vi "Mod_OFDM_DeMapping.vi"(0 "FFT {X}":cdb[][](array[numeric]), 11 "error in (no error)":errorcluster, 13 "Parameters per Ofdm Symbol":T1 {"Data Source"."Data Source"."Register Initial State" format="%08x"}) -> (4 "Bits Out":i8[](array[numeric]), 15 "error out":errorcluster)   [LabVIEW 2010]
uses:
  Controls(Type_DEf)/Parameters per Ofdm Symbol.ctl
  <vilib>/AddOns/Modulation/Digital/General/MT Generate QAM System Parameters(M).vi
  <vilib>/addons/Modulation/Digital/General/MT Map QAM Symbols to Bits.vi
  <vilib>/AddOns/Modulation/Digital/General/MT Generate PSK System Parameters(M).vi
  <vilib>/addons/Modulation/Digital/General/MT Map PSK Symbols to Bits.vi
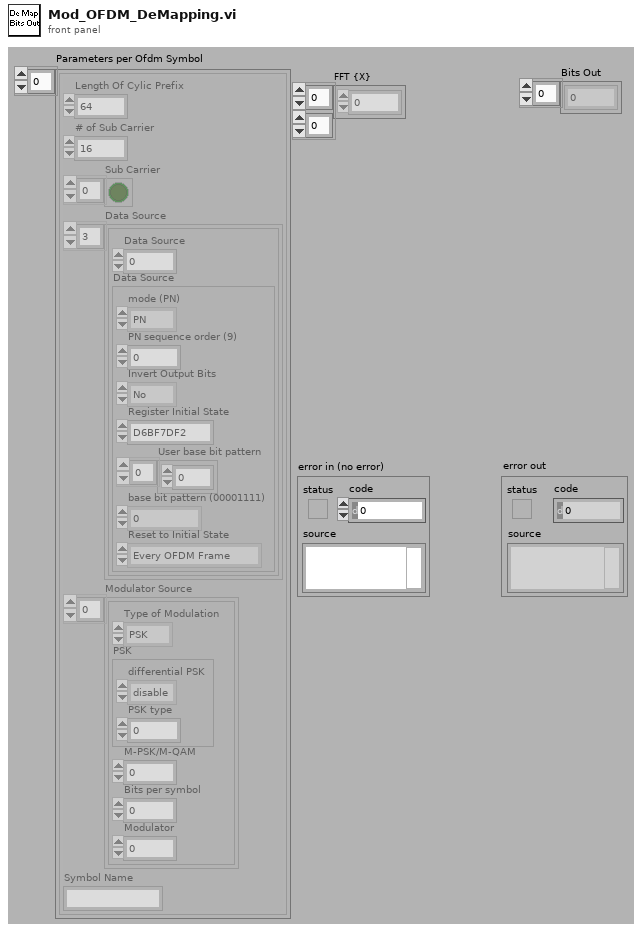
[diagram p1: front panel]
types:
  T1 = typedef "Parameters per Ofdm Symbol.ctl" = cluster{"Length Of Cylic Prefix":i32, "# of Sub Carrier":i32, "Sub Carrier":bool[], "Data Source":cluster{"Data Source":u16, "Data Source":cluster{"mode (PN)":enum16{"PN", "pattern", "user"}, "PN sequence order (9)":i32, "Invert Output Bits":enum16{"No", "Yes"}, "Register Initial State":u32, "User base bit pattern":i8[], "base bit pattern (00001111)":enum16{"0", "1", "01", "0011", "00001111"}, "Reset to Initial State":enum16{"Every OFDM Frame", "Every OFDM Symbol", "Every Sub Carrier"}}}[], "Modulator Source":cluster{"Type of Modulation":enum16{"PSK", "QAM"}, "PSK":cluster{"differential PSK":enum16{"disable", "enable"}, "PSK type":u16}, "M-PSK/M-QAM":i32, "Bits per symbol":i32, "Modulator":u16}[], "Symbol Name":string}[]
  T2 = cluster{"Type of Modulation":enum16{"PSK", "QAM"}, "PSK":cluster{"differential PSK":enum16{"disable", "enable"}, "PSK type":u16}, "M-PSK/M-QAM":i32, "Bits per symbol":i32, "Modulator":u16}[]
  T3 = cluster{"samples per symbol (16)":i32, "symbol map":cdb[]}
  T4 = cluster{"samples per symbol (16)":i32, "symbol map":cdb[], "differential PSK":enum16{"disable", "enable"}, "PSK type":u16}
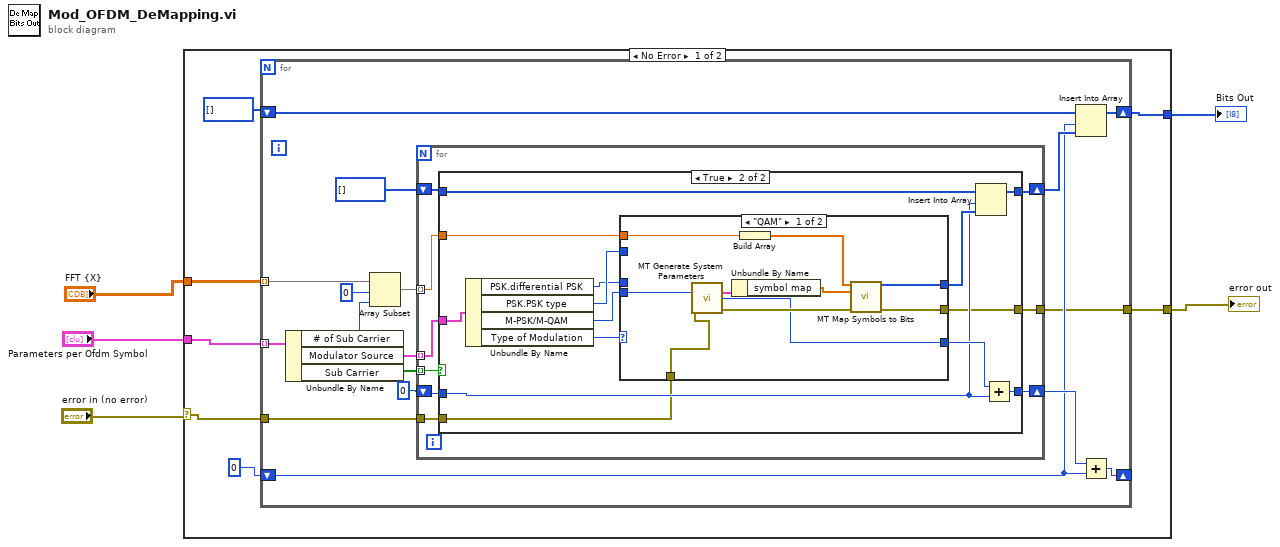
[diagram p0: block diagram]
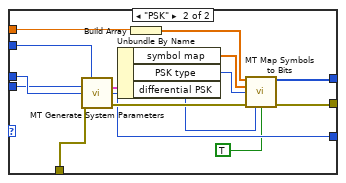
[diagram p3: hidden frame]
diagram:
  n1 = case shown="No Error" "error in (no error)" {
    selector: "error in (no error)" -> [w6 w81]
    tunnel: "Parameters per Ofdm Symbol" -> [w12 _]
    tunnel: "FFT {X}" -> [w11 _]
    tunnel: [w8 _] -> w3
    tunnel: [w7 w81] -> w2
    frame No Error {
      n2 = for {
        tunnel: w12 -> [w29] mode=indexing
        tunnel: w11 -> [w27] mode=indexing
        shift-right: [w21] -> _
        shift-left: 0 -> [w16]
        shift-right: [w19] -> w8
        shift-left: i8[] [] -> [w18]
        tunnel: w6 -> [w14]
        tunnel: [w13] -> w7
        n3 = Unbundle By Name(w29) -> ("# of Sub Carrier"=w28:i32, "Modulator Source"=w24:T2, "Sub Carrier"=w15:bool[])
        n4 = Array Subset(array=w27, index=0, length=w28) -> (w25:cdb[])
        n5 = for {
          tunnel: w25 -> [w36] mode=indexing
          tunnel: w24 -> [w37] mode=indexing
          shift-right: [w33] -> w17
          shift-left: 0 -> [w38]
          shift-right: [w34] -> w20
          shift-left: i8[] [] -> [w35]
          tunnel: w15 -> [w32] mode=indexing
          tunnel: w14 -> [w31]
          tunnel: [w30] -> w13
          n6 = case shown="True" w32 {
            tunnel: w35 -> [w41 w51]
            tunnel: w38 -> [w40 w50]
            tunnel: [w40 w49] -> w33
            tunnel: [w41 w48] -> w34
            tunnel: w37 -> [_ w47]
            tunnel: w36 -> [_ w46]
            tunnel: w31 -> [w39 w43]
            tunnel: [w39 w42] -> w30
            frame False {
            }
            frame True {
              n7 = Unbundle By Name(w47) -> ("PSK.differential PSK"=w54:enum16{"disable", "enable"}, "PSK.PSK type"=w55:u16, "M-PSK/M-QAM"=w45:i32, "Type of Modulation"=w44:enum16{"PSK", "QAM"})
              n8 = case shown="\"QAM\"" w44 {
                tunnel: w46 -> [w63 w78]
                tunnel: w45 -> [w64 w73]
                tunnel: [w61 w77] -> w53
                tunnel: [w60 w74] -> w52
                tunnel: w55 -> [_ w76]
                tunnel: w54 -> [_ w75]
                tunnel: w43 -> [w59 w72]
                tunnel: [w58 w71] -> w42
                frame "QAM" {
                  n9 = call-poly <vilib>:"MT Generate System Parameters.vi"("M-QAM (16)"=w64, "error in (no error)"=w59) -> ("QAM system parameters"=w57:T3, "bits per symbol"=w60:i32, "error out"=w65:errorcluster)  [unwired: 11 in]
                  n10 = Unbundle By Name(w57) -> ("symbol map"=w56:cdb[])
                  n11 = Build Array(w63) -> (w62:cdb[])
                  n12 = call-poly <vilib>:"MT Map Symbols to Bits.vi"("symbols"=w62, "symbol map"=w56, "error in (no error)"=w65) -> ("output bit stream"=w61:i8[], "error out"=w58:errorcluster)  [unwired: 11 in]
                }
                frame "PSK" {
                  n13 = call-poly <vilib>:"MT Generate System Parameters.vi"("PSK type"=w76, "M-PSK (4)"=w73, "differential PSK"=w75, "error in (no error)"=w72) -> ("PSK system parameters"=w70:T4, "bits per symbol"=w74:i32, "error out"=w79:errorcluster)  [unwired: 9 in]
                  n14 = Unbundle By Name(w70) -> ("symbol map"=w69:cdb[], "PSK type"=w68:u16, "differential PSK"=w67:enum16{"disable", "enable"})
                  n15 = Build Array(w78) -> (w80:cdb[])
                  n16 = call-poly <vilib>:"MT Map Symbols to Bits.vi"("symbols"=w80, "symbol map"=w69, "PSK type"=w68, "error in (no error)"=w79, "differential PSK"=w67, "reset? (T)"=TRUE) -> ("output bit stream"=w77:i8[], "error out"=w71:errorcluster)  [unwired: 8 in]
                }
              }
              n17 = Insert Into Array(array=w51, index=w50, new element=w53) -> (w48:i8[])
              n18 = Add(x=w52, y=w50) -> (x+y=w49:i32)
            }
          }
        }
        n19 = Insert Into Array(array=w18, index=w16, new element=w20) -> (w19:i8[])
        n20 = Add(x=w17, y=w16) -> (x+y=w21:i32)
      }
    }
    frame Error {
    }
  }
  "Bits Out" <- w3
  "error out" <- w2
